vi "RT Loop - Analyze Acceleration_queue_2.vi"(7 "testing":bool, 8 "error in (no error)":errorcluster, 9 "Acceleration RT FIFO In":T1, 10 "FPGA VI Reference Out":refnum<k20>, 11 "Message Queue":refnum<queue>) -> (1 "Acceleration RT FIFO Out":T1)   [LabVIEW 2017]
doc: "Read and analyze acceleration waveform data from FPGA via DMA FIFO. If the acceleration is over the limit, then send the acceleration waveform data to the Log Data Loop."
uses:
  UI Error Handlers/support/Message Queue/Message Cluster.ctl
  controls/Acceleration RT FIFO Reference.ctl
  Globals/Global - All RT Loop Stop.vi
  Globals/Global - Configuration Options.vi
  <vilib>/Utility/error.llb/Error Cluster From Error Code.vi
  <vilib>/rvi/errors/niLvFpgaAdjustHostInterfaceError.vi
  <vilib>/rvi/interface/nirviMethod/nirviMethod.xnode
  <vilib>/FPGAPlugInAG/Dynamic/niLvFpga_ReadFifo_Dynamic.vi
  <vilib>/rvi/errors/niLvFpgaMergeErrorWithErrorCode.vi
  UI Error Handlers/support/Logging/Logging.lvlib
  UI Error Handlers/support/Message Queue/Message Queue.lvlib
panel:
  out "AVI Path":path
  out "error out":errorcluster
  out "x-y":u32
  out "G1 status":cluster{"G1 trigger":bool}
  out "G1 status.G1 trigger":bool
  out "sta":bool
  out "logical OR":bool
  in  "Data Rate (Hz)":dbl
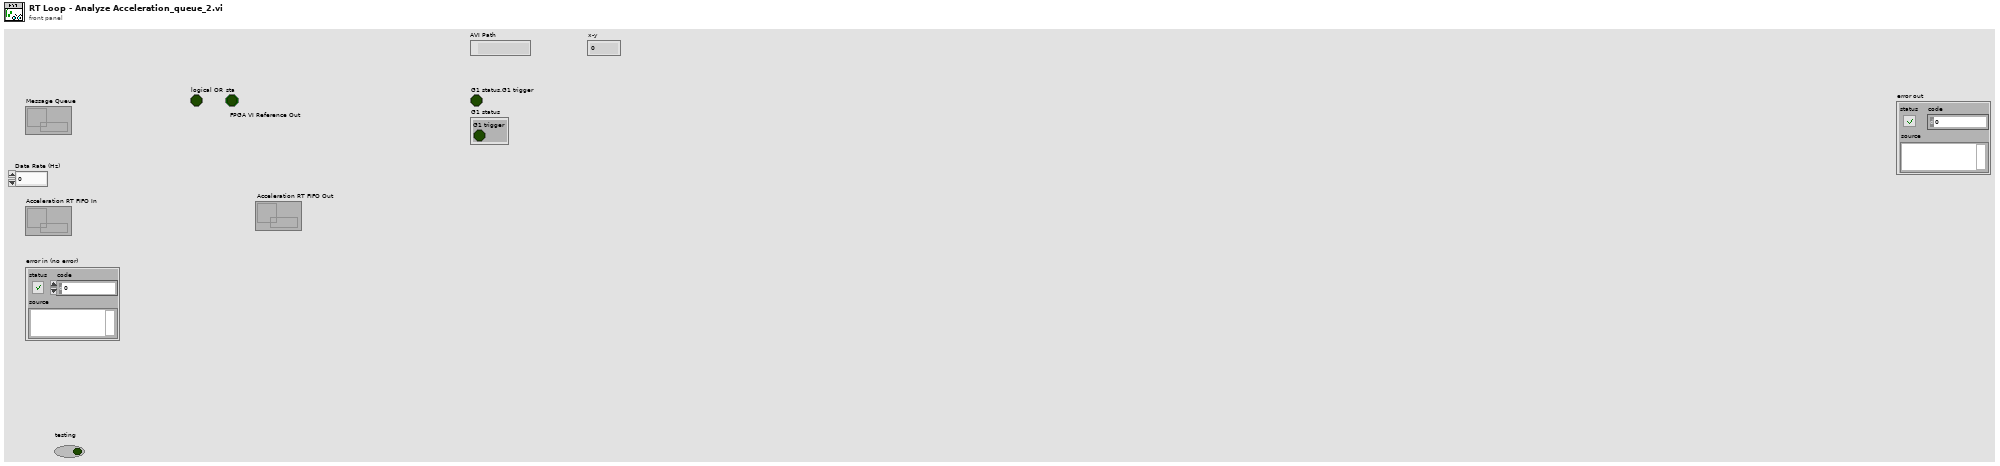
[diagram p1: front panel]
types:
  T1 = typedef "Acceleration RT FIFO Reference.ctl" = refnum<k33>
  T2 = cluster{"Array 2":waveform(dbl)[], "Log File out":refnum<k34>, "AVI Path":path}
  T3 = cluster{"Tool data":cluster{"Number of teeth":sgl}, "Cutting data":cluster{"rpm":sgl}, "Limits":cluster{"Magnitude threshold":sgl, "Tolerance":sgl}, "G1 status":cluster{"G1 trigger":bool}}
  T4 = cluster{waveform(dbl)[], "Log File out":refnum<k34>, "AVI Path":path}
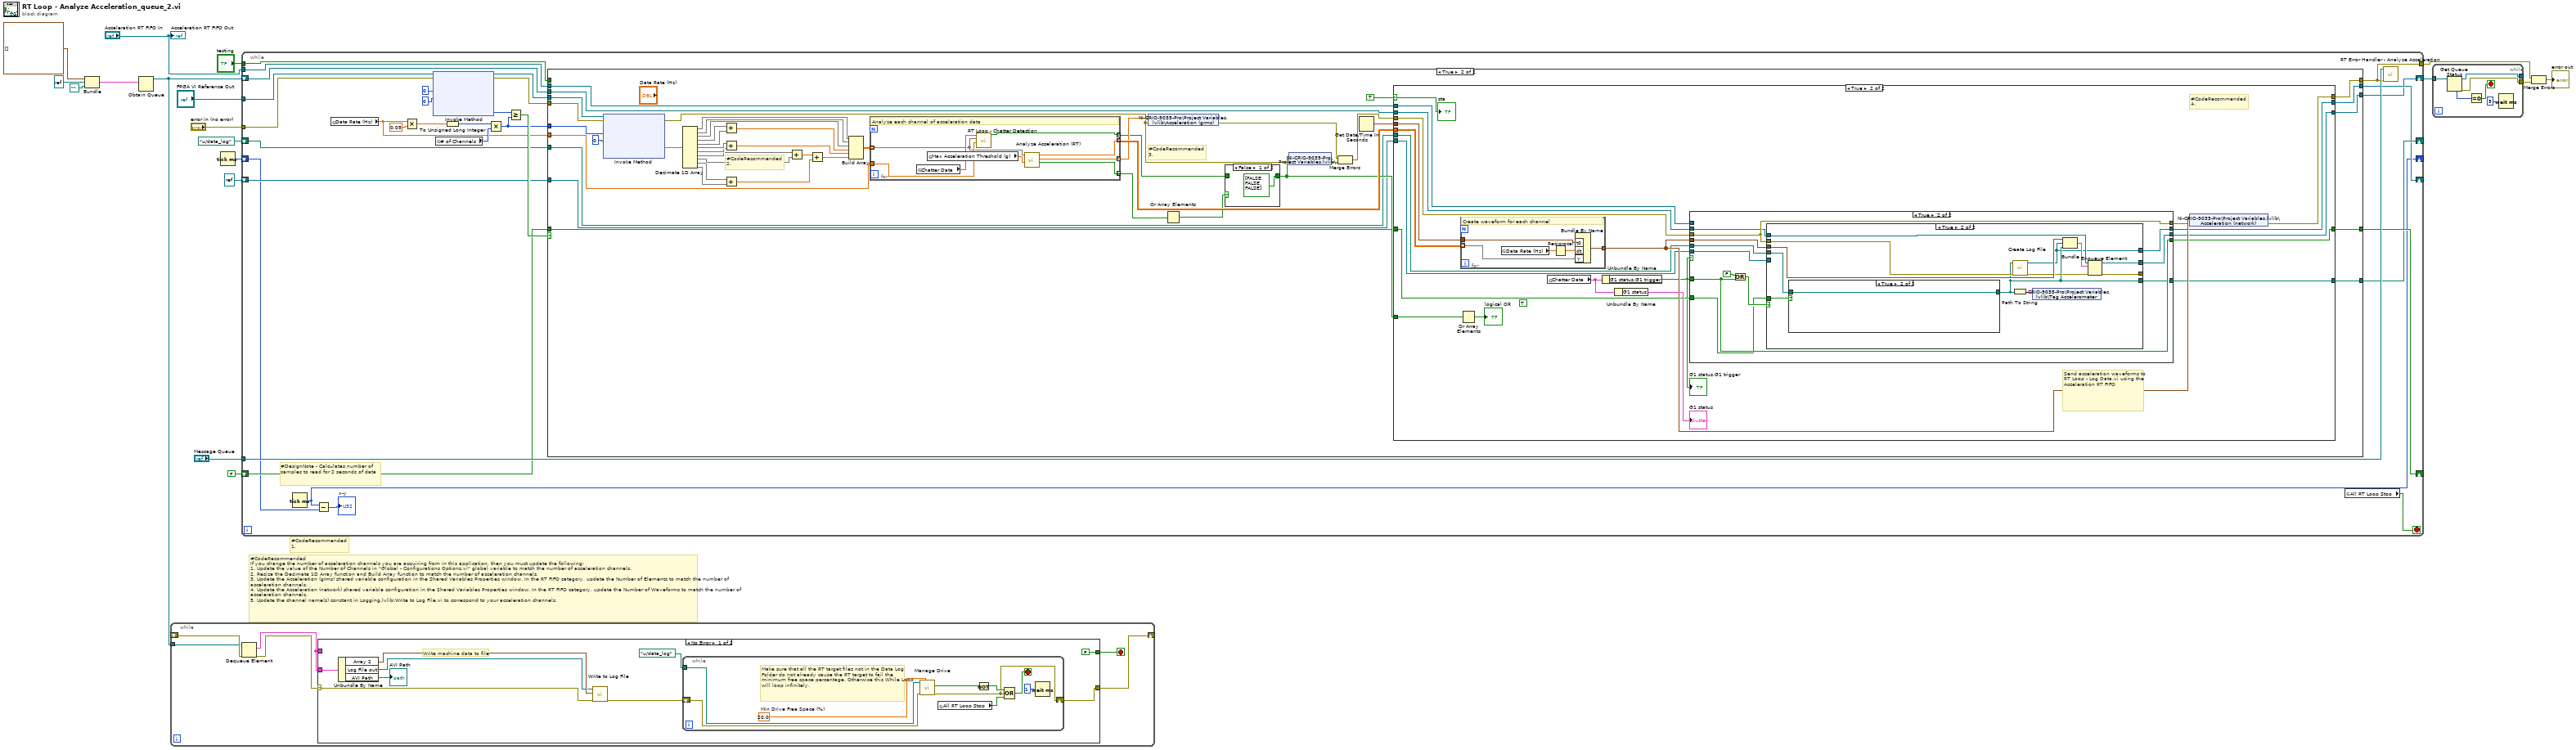
[diagram p0: block diagram]
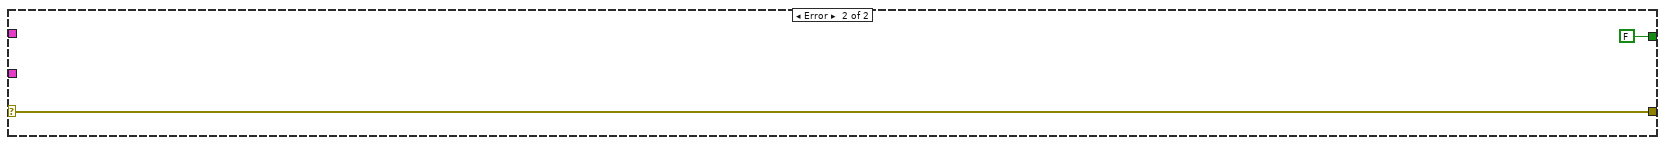
[diagram p2: hidden frame]
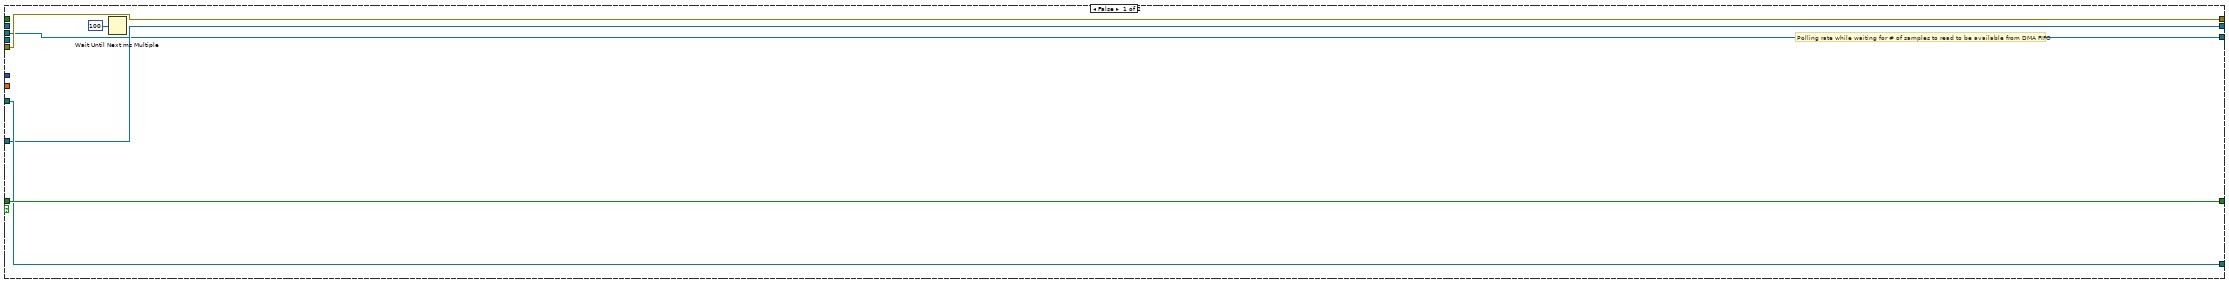
[diagram p3: hidden frame]
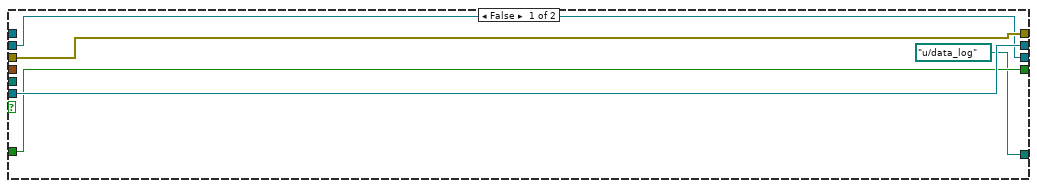
[diagram p6: hidden frame]
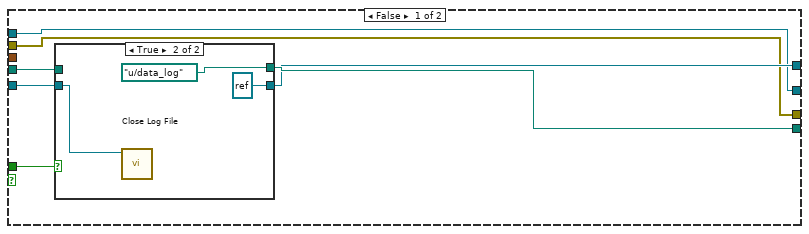
[diagram p7: hidden frame]
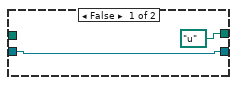
[diagram p8: hidden frame]
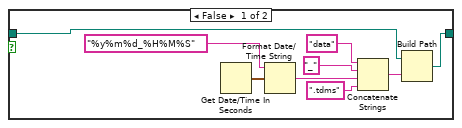
[diagram p9: hidden frame]
diagram:
  # "#CodeRecommended\n1."
  # "#CodeRecommended\nIf you change the number of acceleration channels you are acquiring from in this application, then you must update the following:\n1. Update the value of the Number of Channels in \"Global - Configurations Options.vi\" global variable to match the number of acceleration channels.\n2. Resize the Decimate 1D Array function and Build Array function to match the number of acceleration channels. \n3. Update the Acceleration (grms) shared variable configuration in the Shared Variables Properties window. In the RT FIFO category, update the Number of Elements to match the number of acceleration channels. \n4. Update the Acceleration (network) shared variable configuration in the Shared Variables Properties window. In the RT FIFO category, update the Number of Waveforms to match the number of acceleration channels.\n5. Update the channel name(s) constant in Logging.lvlib:Write to Log File.vi to correspond to your acceleration channels."
  n1 = Bundle("Array 2"=waveform(dbl)[] [], "Log File out"=refnum<k34> refnum, "AVI Path"=path "") -> (w2:T2)  [unwired: 1 in]
  n2 = Obtain Queue(element data type=w2) -> (queue out=w1:refnum<queue>)  [unwired: 4 in, 2 out]
  n3 = while {
    tunnel: w1 -> [w20]
    shift-right: [w21] -> _
    shift-left: _ -> [w24]
    stop <- w22 stop-if-true
    n4 = Dequeue Element(queue=w20, error in (no error)=w24) -> (element=w19:T2, error out=w23:errorcluster)  [unwired: 1 in, 2 out]
    n5 = case shown="No Error" w23 {
      selector: w23 -> [w30 w43]
      tunnel: [FALSE FALSE] -> w22
      tunnel: [w31 w43] -> w21
      tunnel: w19 -> [_ _]
      tunnel: w19 -> [w29 _]
      frame No Error {
        # "Write machine data to file"
        n6 = Unbundle By Name(w29) -> ("Array 2"=w28:waveform(dbl)[], "Log File out"=w27:refnum<k34>, "AVI Path"=→"AVI Path":path)
        n7 = call "Write to Log File.vi"("error in (no error)"=w30, "Array of Waveforms"=w28, "Log File in"=w27) -> ("error out"=w26:errorcluster)  [unwired: 7 in, 1 out]
        n8 = while {
          shift-right: [w37] -> w31
          shift-left: w26 -> [w38]
          tunnel: path "u:/data_log" ("AVI Path") -> [w35]
          stop <- w42 stop-if-true
          w36 = 20.0  # Min Drive Free Space (%)
          # "Make sure that all the RT target files not in the Data Log Folder do not already cause the RT target to fail the minimum free space percentage. Otherwise this While Loop will loop infinitely."
          n9 = call "Manage Drive.vi"("Min Drive Free Space (%)"=w36, "error in"=w38, "Data Folder"=w35) -> ("error out"=w37:errorcluster, "Drive Space Below Limit"=w34:bool)  [unwired: 7 in]
          n10 = global read "Global - All RT Loop Stop.vi" "All RT Loop Stop"() -> (w39:bool)
          n11 = Not(x=w34) -> (.not. x?=w41:bool)
          n12 = Compound Arithmetic op=OR(w41, w37, w39) -> (w42:bool)
          n13 = Wait (ms)(milliseconds to wait=u32 1) -> ()  [unwired: 1 out]
        }
      }
      frame Error {
      }
    }
  }
  n14 = Tick Count (ms)() -> (millisecond timer value=w10:u32)
  n15 = while {
    tunnel: "FPGA VI Reference Out" -> [w74]
    tunnel: "error in (no error)" -> [w73]
    tunnel: "Message Queue" -> [w66]
    tunnel: "Acceleration RT FIFO In" -> [w65]
    tunnel: "testing" -> [w57]
    shift-right: [w54] -> _
    shift-left: path "u:/data_log" ("AVI Path") -> [w53]
    shift-right: [w56] -> _
    shift-left: FALSE -> [w55]
    shift-right: [w52] -> _
    shift-left: refnum<k34> refnum ("Log File out") -> [w51]
    shift-right: [w49] -> _
    shift-left: w10 -> [w50]
    shift-right: [w45] -> w3
    shift-left: w1 -> [w47]
    tunnel: [w46] -> w5
    stop <- w67 stop-if-true
    # "#DesignNote - Calculates number of samples to read for 2 seconds of data"
    n16 = Tick Count (ms)() -> (millisecond timer value=w49:u32)
    n17 = Subtract(x=w49, y=w50) -> (x-y=→"x-y":u32)
    n18 = global read "Global - Configuration Options.vi" "Data Rate (Hz)"() -> (w59:dbl)
    n19 = Multiply(x=w59, y=0.05) -> (x*y=w63:dbl)
    n20 = xnode "Invoke Method"("FPGA VI Reference In"=w74, "error in"=w73, "Number of Elements"=u32 0, "Timeout (ms)"=0) -> ("FPGA VI Reference Out"=w70:refnum<k20>, "error out"=w69:errorcluster, "Elements Remaining"=w58:u32)  [unwired: 1 out]
    n21 = global read "Global - Configuration Options.vi" "# of Channels"() -> (w60:u32)
    n22 = To Unsigned Long Integer(number=w63) -> (unsigned 32bit integer=w62:u32)
    n23 = Multiply(x=w62, y=w60) -> (x*y=w61:u32)
    n24 = Greater Or Equal?(x=w58, y=w61) -> (x >= y?=w68:bool)
    n25 = case shown="True" w68 {
      tunnel: w70 -> [_ w125]
      tunnel: w69 -> [w80 w124]
      tunnel: [w80 w120] -> w46
      tunnel: w61 -> [_ w123]
      tunnel: w65 -> [_ w118]
      tunnel: w59 -> [_ w114]
      tunnel: w57 -> [_ _]
      tunnel: [w78 w106] -> w56
      tunnel: w55 -> [w78 w105]
      tunnel: [w77 w104] -> w54
      tunnel: w53 -> [w77 w103]
      tunnel: [w76 w102] -> w52
      tunnel: w51 -> [w76 w101]
      tunnel: w47 -> [w75 w82]
      tunnel: [w75 w81] -> w45
      frame False {
        # "Polling rate while waiting for # of samples to read to be available from DMA FIFO"
        n26 = Wait Until Next ms Multiple(millisecond multiple=u32 100) -> ()  [unwired: 1 out]
      }
      frame True {
        # "#CodeRecommended\n3."
        # "#CodeRecommended\n2."
        n27 = xnode "Invoke Method"("FPGA VI Reference In"=w125, "error in"=w124, "Number of Elements"=w123, "Timeout (ms)"=0) -> ("error out"=w113:errorcluster, "Data"=w117:sgl[])  [unwired: 2 out]
        n28 = Decimate 1D Array(w117) -> (w98:sgl[], w97:sgl[], w96:sgl[], w95:sgl[], w94:sgl[], w92:sgl[], w91:sgl[], w90:sgl[], w89:sgl[], w88:sgl[], w87:sgl[])
        n29 = Add(x=w95, y=w94) -> (x+y=w93:sgl[])
        n30 = Add(x=w92, y=w91) -> (x+y=w83:sgl[])
        n31 = Add(x=w88, y=w87) -> (x+y=w85:sgl[])
        n32 = Add(x=w90, y=w89) -> (x+y=w86:sgl[])
        n33 = Add(x=w86, y=w85) -> (x+y=w84:sgl[])
        n34 = Build Array(w98, w97, w96, w93, w83, w84) -> (w99:sgl[][])
        n35 = for {
          tunnel: [w135] -> w119 mode=indexing
          tunnel: [w134] -> w116 mode=indexing
          tunnel: [w133] -> w115 mode=indexing
          tunnel: w114 -> [w131]
          tunnel: [w130] -> w108 mode=indexing
          tunnel: w99 -> [w128] mode=indexing
          # "Analyze each channel of acceleration data"
          n36 = global read "Global - Configuration Options.vi" "Chatter Data"() -> (w129:T3)
          n37 = global read "Global - Configuration Options.vi" "Max Acceleration Threshold (g)"() -> (w132:sgl)
          n38 = call "RT Loop - Chatter Detection.vi"("Data Rate (Hz)"=w131, "Acceleration Waveform (SGL)"=w128, "Chatter Data"=w129) -> ("Chatter?"=w130:bool)  [unwired: 8 in]
          n39 = call "Analyze Acceleration (RT).vi"("Max Instantaneous Acceleration (g)"=w132, "Acceleration Waveform (SGL)"=w128) -> ("Over Limit?"=w135:bool, "Acceleration (grms)"=w133:dbl, "Acceleration Waveform (DBL)"=w134:dbl[])  [unwired: 7 in]
        }
        n40 = shared-variable "NI-CRIO-9035-Pro\\Project Variables.lvlib\\Acceleration (grms)"(w115, error in=w113) -> (error out=w111:errorcluster)
        n41 = Or Array Elements(Boolean array=w119) -> (logical OR=w109:bool)
        n42 = case shown="False" w109 {
          tunnel: w108 -> [_ w127]
          tunnel: [bool[] [FALSE, FALSE, FALSE] ("Chatter?") w127] -> w107
          frame False {
          }
          frame True {
          }
        }
        n43 = shared-variable "NI-CRIO-9035-Pro\\Project Variables.lvlib\\Chatter?"(w107, error in=w113) -> (error out=w112:errorcluster)
        n44 = Merge Errors(w111, w112) -> (w110:errorcluster)
        n45 = Get Date/Time In Seconds() -> (seconds since 1Jan1904=w121:timestamp)
        n46 = case shown="True" TRUE {
          selector: TRUE -> [_ w153]
          tunnel: w121 -> [_ w161]
          tunnel: w110 -> [w140 w160]
          tunnel: [w140 w159] -> w120
          tunnel: w118 -> [_ w157]
          tunnel: w116 -> [_ w156]
          tunnel: w107 -> [_ w154]
          tunnel: [w139 w150] -> w106
          tunnel: w105 -> [w139 w149]
          tunnel: [w138 w148] -> w104
          tunnel: w103 -> [w138 w143]
          tunnel: [w137 w147] -> w102
          tunnel: w101 -> [w137 w146]
          tunnel: w82 -> [w136 w142]
          tunnel: [w136 w141] -> w81
          frame False {
          }
          frame True {
            (unwired) TRUE
            # "#CodeRecommended\n4."
            # "Send acceleration waveforms to RT Loop - Log Data.vi using the Acceleration RT FIFO"
            n47 = for {
              tunnel: w156 -> [w217] mode=indexing
              tunnel: w161 -> [w216]
              tunnel: [w214] -> w158 mode=indexing
              # "Create waveform for each channel"
              n48 = global read "Global - Configuration Options.vi" "Data Rate (Hz)"() -> (w213:dbl)
              n49 = Reciprocal(x=w213) -> (1/x=w215:dbl)
              n50 = Bundle By Name("t0"=w216, "dt"=w215, "Y"=w217) -> (w214:waveform(dbl))  [unwired: 1 in]
            }
            n51 = Or Array Elements(Boolean array=w154) -> (logical OR=→"logical OR":bool)
            n52 = global read "Global - Configuration Options.vi" "Chatter Data"() -> (w152:T3)
            n53 = Unbundle By Name(w152) -> ("G1 status.G1 trigger"=w144:bool)
            "G1 status.G1 trigger" <- w144
            n54 = Unbundle By Name(w152) -> ("G1 status"=→"G1 status":cluster{"G1 trigger":bool})
            n55 = case shown="True" w144 {
              tunnel: w160 -> [w166 w169]
              tunnel: w158 -> [_ w170]
              tunnel: w157 -> [_ _]
              tunnel: w144 -> [w164 w176]
              tunnel: [w164 w176] -> w150
              tunnel: w149 -> [_ w175]
              tunnel: [path "u:/data_log" ("AVI Path") w174] -> w148
              tunnel: w143 -> [_ w173]
              tunnel: [w165 w172] -> w147
              tunnel: w146 -> [w165 w171]
              tunnel: [w166 w169] -> w145
              tunnel: w142 -> [w162 w168]
              tunnel: [w162 w167] -> w141
              frame False {
              }
              frame True {
                n56 = Or(x=FALSE, y=w176) -> (x .or. y?=w178:bool)
                n57 = case shown="True" w178 {
                  tunnel: w173 -> [w182 w202]
                  tunnel: [w185 w196] -> w174
                  tunnel: w175 -> [w183 w201]
                  tunnel: w171 -> [w184 _]
                  tunnel: w170 -> [_ w197]
                  tunnel: [w181 w193] -> w172
                  tunnel: w169 -> [w180 w199]
                  tunnel: [w180 w191] -> _
                  tunnel: w168 -> [w179 w198]
                  tunnel: [w179 w194] -> w167
                  frame False {
                    n58 = case shown="True" w183 {
                      tunnel: [path "u:/" ("AVI Path") path "u:/data_log" ("AVI Path")] -> w185
                      tunnel: w184 -> [w186 w189]
                      tunnel: w182 -> [_ _]
                      tunnel: [w186 refnum<k34> refnum ("Log File out")] -> w181
                      frame False {
                      }
                      frame True {
                        n59 = call "Close Log File.vi"("tdms file"=w189) -> ()  [unwired: 10 in, 1 out]
                      }
                    }
                  }
                  frame True {
                    n60 = case shown="True" w201 {
                      tunnel: w202 -> [w204 w212]
                      tunnel: [w203 w212] -> w196
                      frame False {
                        n61 = Get Date/Time In Seconds() -> (seconds since 1Jan1904=w207:timestamp)
                        n62 = Format Date/Time String(time format string (%c)="%y%m%d_%H%M%S", seconds (now)=w207) -> (date/time string=w210:string)  [unwired: 1 out]
                        n63 = Concatenate Strings("data" ("string"), "_" ("string"), w210, ".tdms" ("string")) -> (w205:string)
                        n64 = Build Path(base path=w204, name or relative path=w205) -> (appended path=w203:path)
                      }
                      frame True {
                      }
                    }
                    n65 = Path To String(path=w196) -> (string=w200:string)
                    n66 = call "Create Log File.vi"("error in (no error)"=w199, "Acceleration Exceeded Log Folder"=w196) -> ("error out"=w192:errorcluster, "Log File out"=w193:refnum<k34>)  [unwired: 8 in]
                    n67 = shared-variable "NI-CRIO-9035-Pro\\Project Variables.lvlib\\Tag Accelerometer"(w200) -> ()  [unwired: 1 in, 1 out]
                    n68 = Bundle(w197, "Log File out"=w193, "AVI Path"=w196) -> (w195:T4)  [unwired: 1 in]
                    n69 = Enqueue Element(queue=w198, element=w195, error in (no error)=w192) -> (queue out=w194:refnum<queue>, error out=w191:errorcluster)  [unwired: 1 in, 1 out]
                  }
                }
              }
            }
            n70 = shared-variable "NI-CRIO-9035-Pro\\Project Variables.lvlib\\Acceleration (network)"(w158, error in=w145) -> (error out=w159:errorcluster)
            "sta" <- w153
          }
        }
      }
    }
    n71 = global read "Global - All RT Loop Stop.vi" "All RT Loop Stop"() -> (w67:bool)
    n72 = call "RT Error Handler - Analyze Acceleration.vi"("error in (no error)"=w46, "Message Queue"=w66) -> ()  [unwired: 9 in, 1 out]
  }
  n73 = while {
    tunnel: [w222] -> w4
    tunnel: [w220] -> _
    tunnel: w3 -> [w218]
    stop <- w221 stop-if-true
    n74 = Get Queue Status(queue=w218) -> (queue out=w220:refnum<queue>, error out=w222:errorcluster, # elements in queue=w219:i32)  [unwired: 2 in, 5 out]
    n75 = Equal To 0?(x=w219) -> (x = 0?=w221:bool)
    n76 = Wait (ms)(milliseconds to wait=u32 5) -> ()  [unwired: 1 out]
  }
  n77 = Merge Errors(w5, w4) -> (→"error out":errorcluster)
  "Acceleration RT FIFO Out" <- "Acceleration RT FIFO In"
